vi "Execute.vi"(8 "Error In":errorcluster, 11 "Central Message Handler In":refnum<class "Central Message Handler.lvclass">) -> (0 "Error Out":errorcluster, 3 "Central Message Handler Out":refnum<class "Central Message Handler.lvclass">)   [LabVIEW 2021, in "Central Message Handler.lvclass"]
uses:
  Central Message Handler.lvclass
  Process/Public/Controls/Process Message.ctl
  Accessors/Central Message Handler Queue/Get Central Message Handler Queue.vi
  Accessors/Processes Queues Map/Get Processes Queues Map.vi
  Process/Process.lvclass
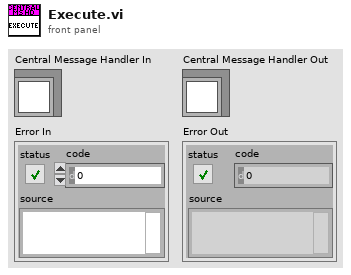
[diagram p1: front panel]
types:
  T1 = typedef "Process.lvclass/Process Message.ctl" = cluster{"Command":string, "Data":variant}
  T2 = typedef "Central Message Handler.lvclass/Message.ctl" = cluster{"Command":string, "Data":variant, "Receiver":string}
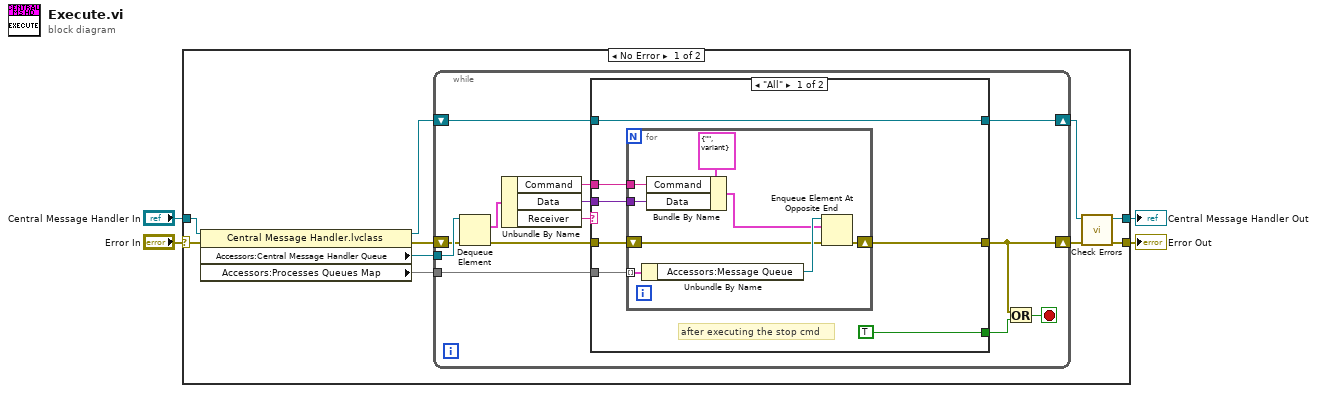
[diagram p0: block diagram]
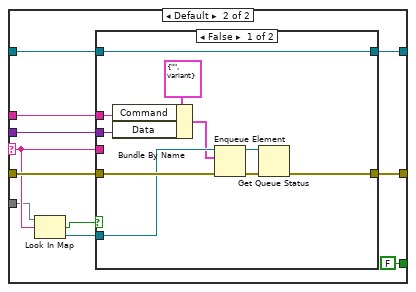
[diagram p2: hidden frame]
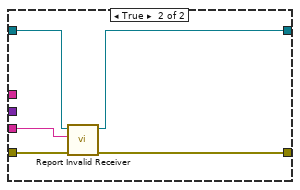
[diagram p3: hidden frame]
diagram:
  n1 = case shown="No Error" "Error In" {
    selector: "Error In" -> [w14 w70]
    tunnel: [w5 w70] -> w3
    tunnel: "Central Message Handler In" -> [w13 w69]
    tunnel: [w6 w69] -> w1
    frame No Error {
      n2 = property class="Central Message Handler.lvclass"(reference=w13, error in=w14) -> (reference out=w9:refnum<class "Central Message Handler.lvclass">, error out=w11:errorcluster, "Accessors:Central Message Handler Queue"=w12:refnum<queue>, "Accessors:Processes Queues Map"=w10:map{string, refnum<queue>})
      n3 = while {
        tunnel: w12 -> [w27]
        shift-right: [w19] -> w8
        shift-left: w11 -> [w26]
        tunnel: w10 -> [w24]
        shift-right: [w15] -> w7
        shift-left: w9 -> [w16]
        stop <- w17 stop-if-true
        n4 = Dequeue Element(queue=w27, error in (no error)=w26) -> (element=w25:T2, error out=w22:errorcluster)  [unwired: 1 in, 2 out]
        n5 = Unbundle By Name(w25) -> ("Command"=w21:string, "Data"=w20:variant, "Receiver"=w23:string)
        n6 = case shown="\"All\"" w23 {
          selector: w23 -> [_ w48]
          tunnel: w24 -> [w33 w45]
          tunnel: w22 -> [w32 w53]
          tunnel: w21 -> [w31 w51]
          tunnel: w20 -> [w30 w50]
          tunnel: [TRUE FALSE] -> w18
          tunnel: [w29 w47] -> w19
          tunnel: w16 -> [w28 w44]
          tunnel: [w28 w43] -> w15
          frame "All" {
            # "after executing the stop cmd"
            n7 = for {
              tunnel: w33 -> [w42] mode=indexing
              tunnel: w31 -> [w38]
              tunnel: w30 -> [w37]
              shift-right: [w35] -> w29
              shift-left: w32 -> [w40]
              n8 = Unbundle By Name(w42) -> ("Accessors:Message Queue"=w41:refnum<queue>)
              n9 = Bundle By Name(cluster=T1 {"Command"="", "Data"=variant} ("element"), "Command"=w38, "Data"=w37) -> (w36:T1)
              n10 = Enqueue Element At Opposite End(queue=w41, element=w36, error in (no error)=w40) -> (error out=w35:errorcluster)  [unwired: 1 in, 2 out]
            }
          }
          frame Default {
            n11 = Look In Map(map=w45, key=w48) -> (key not found?=w49:bool, value=w52:refnum<queue>)  [unwired: 1 in]
            n12 = case shown="False" w49 {
              tunnel: w53 -> [w63 w68]
              tunnel: w52 -> [w62 _]
              tunnel: w51 -> [w60 _]
              tunnel: w50 -> [w59 _]
              tunnel: w48 -> [_ w66]
              tunnel: [w56 w67] -> w47
              tunnel: w44 -> [w57 w65]
              tunnel: [w57 w64] -> w43
              frame False {
                n13 = Bundle By Name(cluster=T1 {"Command"="", "Data"=variant} ("element"), "Command"=w60, "Data"=w59) -> (w58:T1)
                n14 = Enqueue Element(queue=w62, element=w58, error in (no error)=w63) -> (queue out=w54:refnum<queue>, error out=w55:errorcluster)  [unwired: 1 in, 1 out]
                n15 = Get Queue Status(queue=w54, error in (no error)=w55) -> (error out=w56:errorcluster)  [unwired: 1 in, 7 out]
              }
              frame True {
                n16 = call "Report Invalid Receiver.vi"("Error In"=w68, "Receiver"=w66, "Central Message Handler In"=w65) -> ("Error Out"=w67:errorcluster, "Central Message Handler Out"=w64:refnum<class "Central Message Handler.lvclass">)  [unwired: 7 in]
              }
            }
          }
        }
        n17 = Or(x=w19, y=w18) -> (x .or. y?=w17:bool)
      }
      n18 = call "Check Errors.vi"("Error In"=w8, "Central Message Handler In"=w7) -> ("Error Out"=w5:errorcluster, "Central Message Handler Out"=w6:refnum<class "Central Message Handler.lvclass">)  [unwired: 8 in]
    }
    frame Error {
    }
  }
  "Central Message Handler Out" <- w1
  "Error Out" <- w3
